vi "QMH_Change_CurrentStatus.vi"(0 "Status array in":T1=[TRUE, FALSE, FALSE, FALSE, FALSE, FALSE], 5 "Array - String":string[](array[string])=["Template #1", "Template #2", "Filter Wheel", "Live"], 7 "String to find":string="Template #2", 9 "New status":bool=TRUE, 11 "error in (no error)":errorcluster) -> (4 "Status array out":T1=[TRUE, FALSE, FALSE, FALSE, FALSE, FALSE], 15 "error out":errorcluster)   [LabVIEW 2021]
doc: "This Vi changes the status of a specific task corresponding to the string and the boolean inputs."
uses:
  Controls/Control 2.ctl
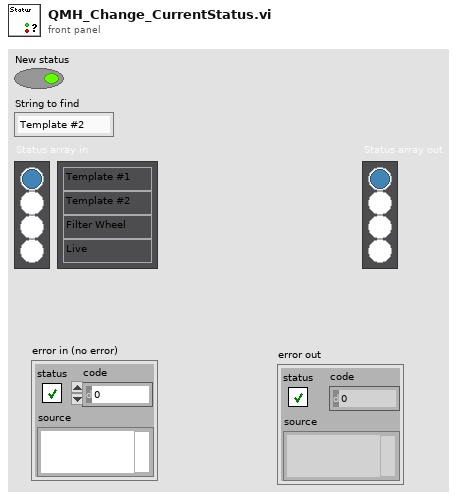
[diagram p1: front panel]
types:
  T1 = typedef "Control 2.ctl" = bool[]
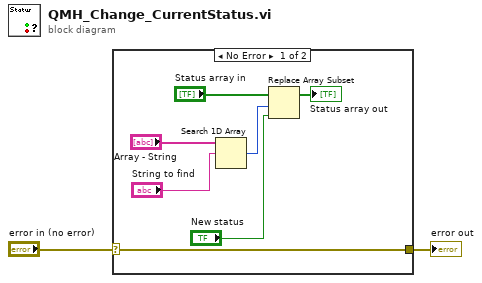
[diagram p0: block diagram]
diagram:
  n1 = case shown="No Error" "error in (no error)" {
    selector: "error in (no error)" -> [w4 w10]
    tunnel: [w4 w10] -> w2
    frame No Error {
      n2 = Search 1D Array(1D array="Array - String", element="String to find") -> (index of element=w6:i32)  [unwired: 1 in]
      n3 = Replace Array Subset(array="Status array in", new element="New status", index=w6) -> (→"Status array out":T1)
    }
    frame Error {
    }
  }
  "error out" <- w2
